vi "AO Update Channel (single-point waveform).vi"(0 "value":waveform(dbl)={"t0"=timestamp(0 s since 1904-01-01), "dt"=0.0, "Y"=[]}, 1 "channel (0)":tag="0", 2 "device":i16=1) -> ()   [LabVIEW 2009]
doc: "Generates a timed, simple-buffered waveform for the given output channel at the specified update rate."
uses:
  <vilib>/Daq/ao.llb/AO Write One Update (single-point waveform).vi
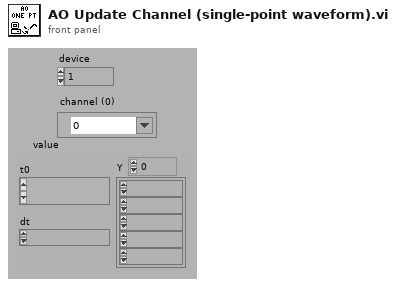
[diagram p1: front panel]
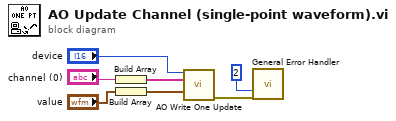
[diagram p0: block diagram]
diagram:
  n1 = Build Array("channel (0)") -> (w6:tag[])
  n2 = Build Array("value") -> (w5:waveform(dbl)[])
  n3 = call-poly <vilib>:"AO Write One Update.vi"("device (1)"="device", "channels (0)"=w6, "waveform data"=w5) -> ("error out"=w2:errorcluster)  [unwired: 12 in]
  n4 = call <vilib>:"General Error Handler.vi"("type of dialog (OK msg:1)"=u16 2, "error in (no error)"=w2) -> ()  [unwired: 9 in, 5 out]
